vi "Select Channels Dialog.vi"(7 "Channel Label":string="System Channels", 8 "error in (no error)":errorcluster, 9 "Custom Filter":refnum<k24>, 10 "Filter":u8(ring)=1 items=["K_CHAN_R", "K_CHAN_W", "K_CHAN_RW", "K_CHAN_VOLT", "K_CHAN_FAULT", "K_ALL", "K_CUSTOM"], 11 "Start Item Ref":T1=18446744073709551615 format="%.0x") -> (0 "error out":errorcluster, 1 "Canceled":bool, 3 "Channels":string[](array[string]))   [LabVIEW 2013, in "Datadashboard CD Custom Device.lvlib"]
uses:
  Datadashboard CD Custom Device.lvlib
  <vilib>/NI Veristand/Custom Device API/Custom Device Item Ref.ctl
  NationalInstruments.VeriStand.SystemStorageUI
  NationalInstruments.VeriStand.SystemStorage
  <vilib>/NI Veristand/Custom Device API/Custom Device API.lvlib
panel:
  in  "OK":bool
  in  "Cancel":bool
  in  "TreeBrowserWF":refnum<k24>(container)
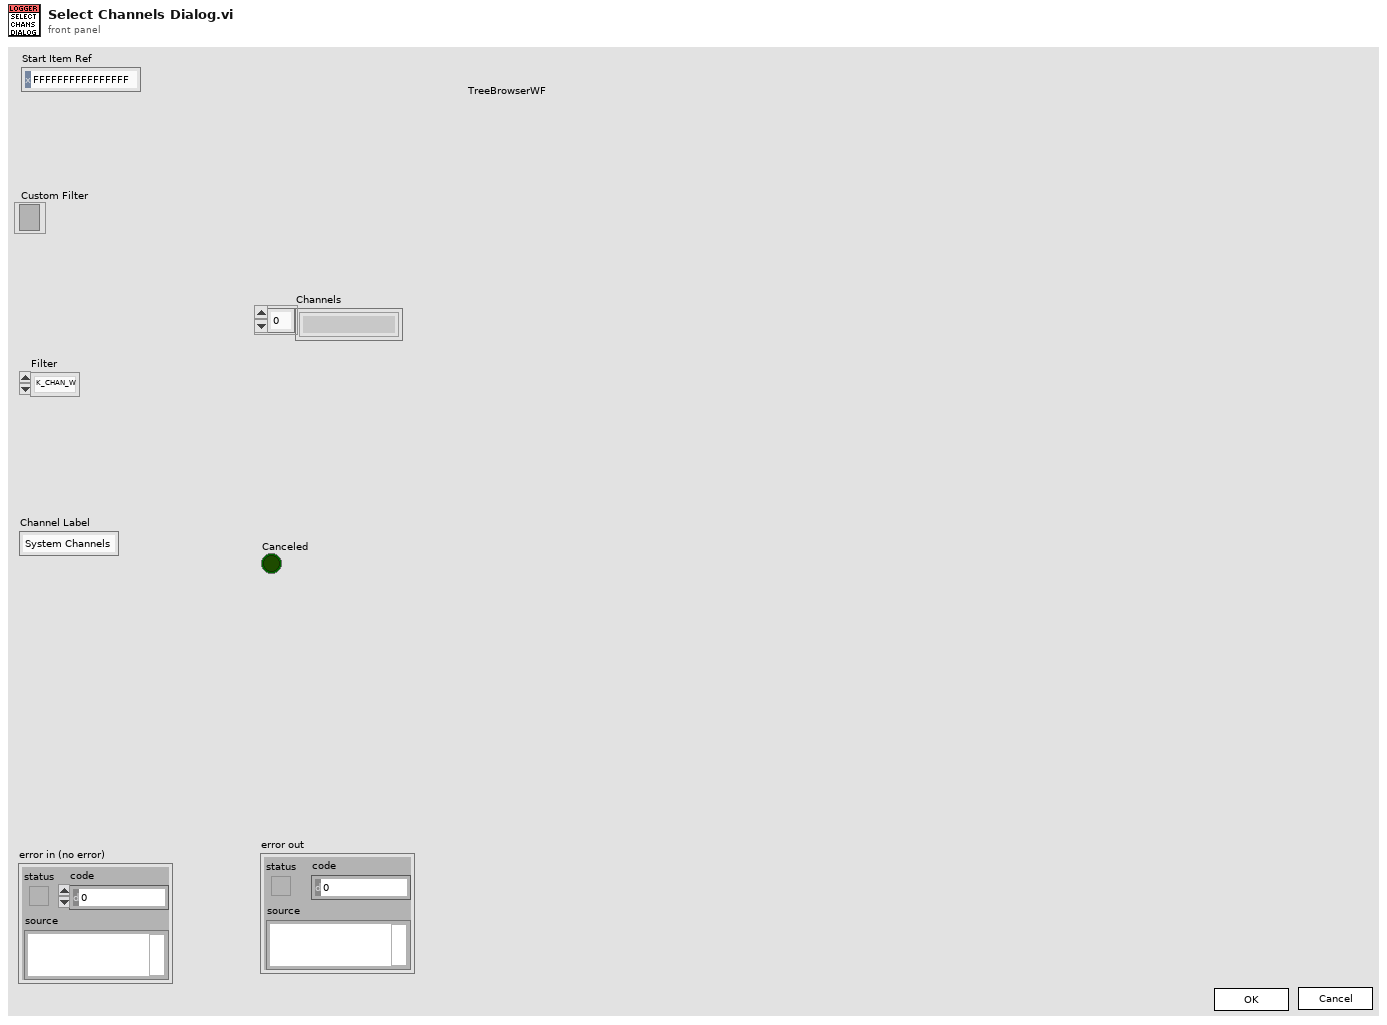
[diagram p1: front panel]
types:
  T1 = typedef "Custom Device API.lvlib/Custom Device Item Ref.ctl" = u64
  T2 = cluster{"Shut Down":bool, "Error":errorcluster, "Root":refnum<k24>, "Cancel":bool, "MapTree":cluster{"Ref":refnum<k24>, "Filter":refnum<k24>}, "Channels":string[]}
  T3 = typedef "Custom Device API.lvlib/Custom Device Pointer.ctl" = refnum<k24>
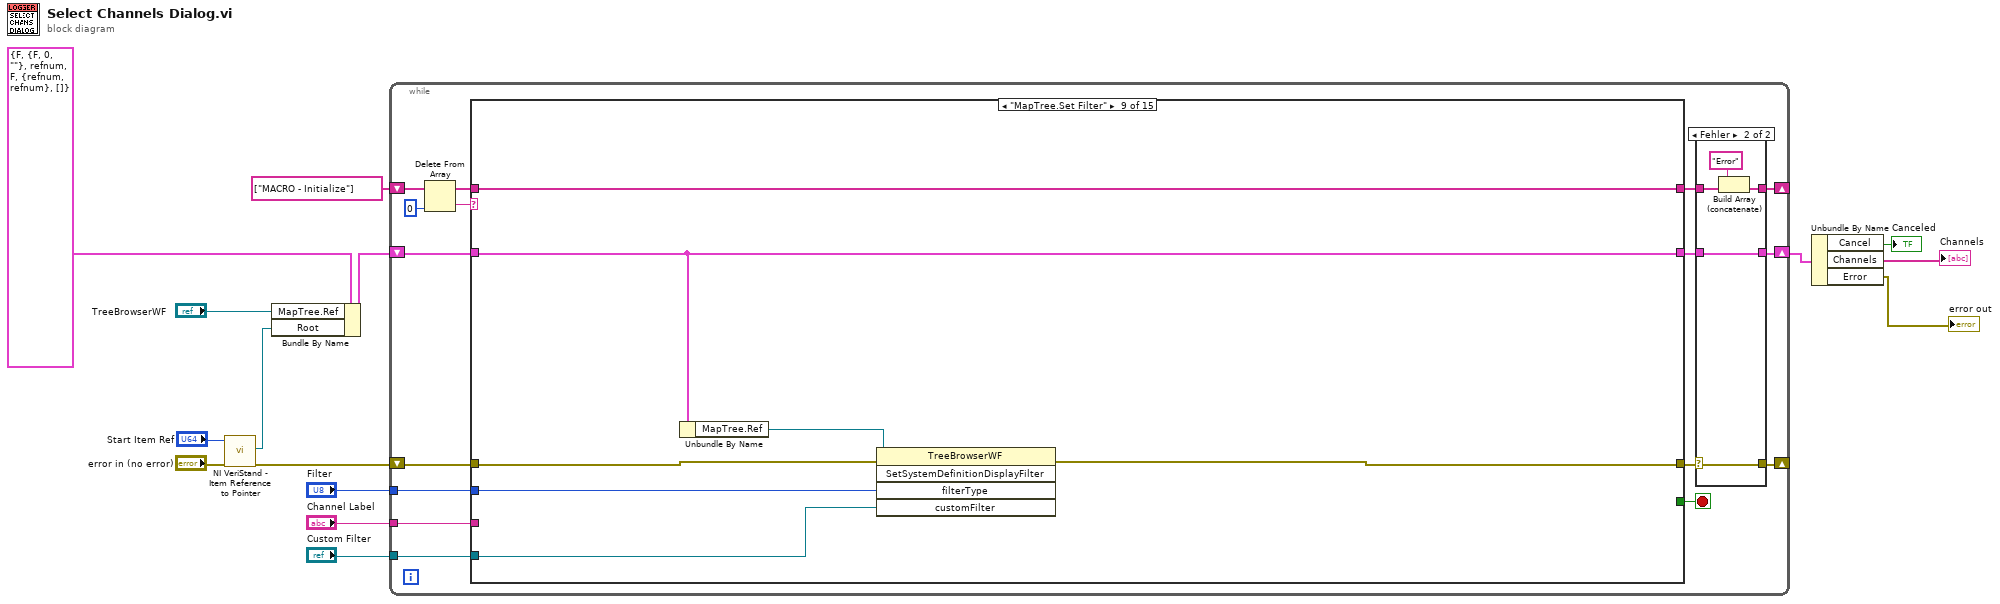
[diagram p0: block diagram]
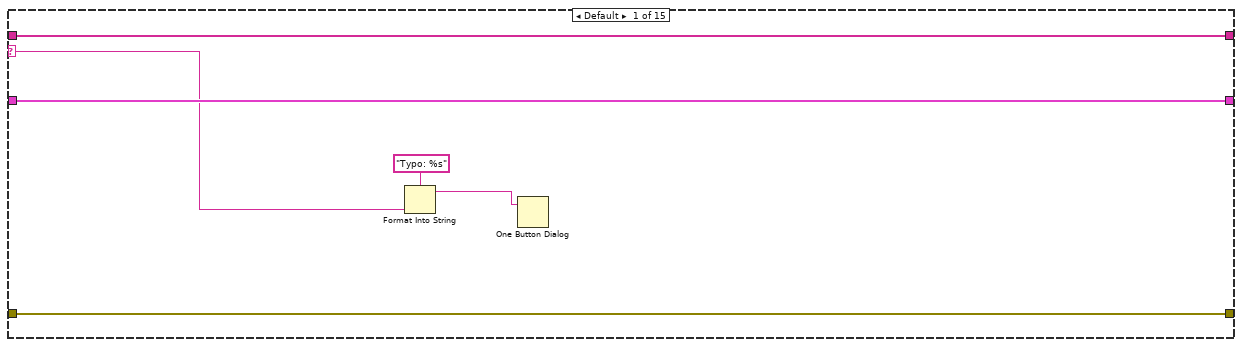
[diagram p3: hidden frame]
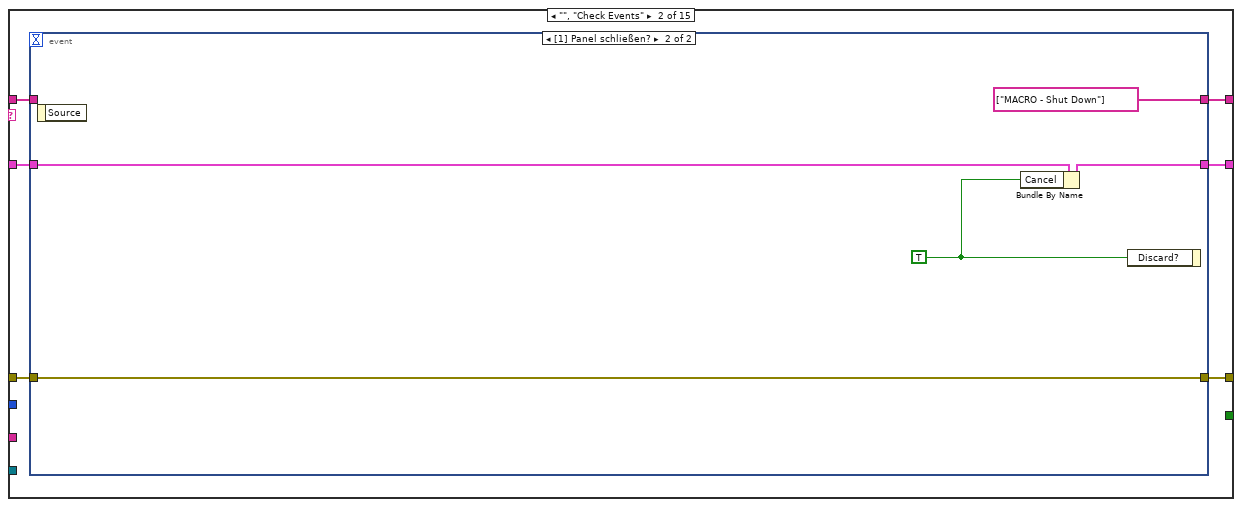
[diagram p4: hidden frame]
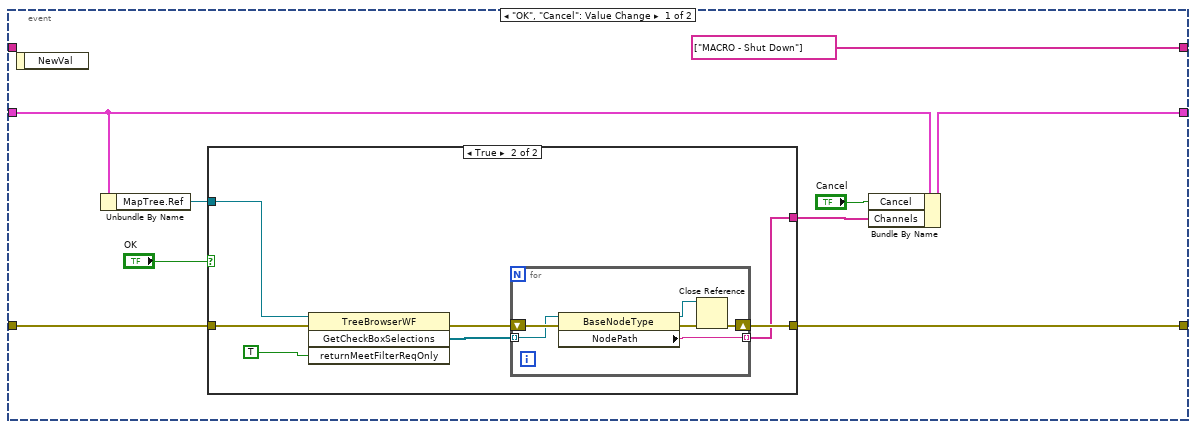
[diagram p5: hidden frame]
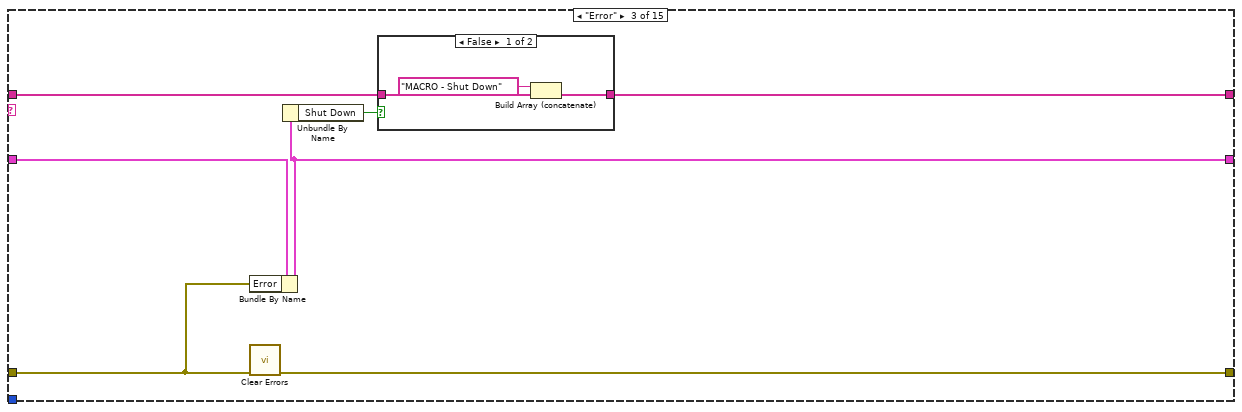
[diagram p7: hidden frame]
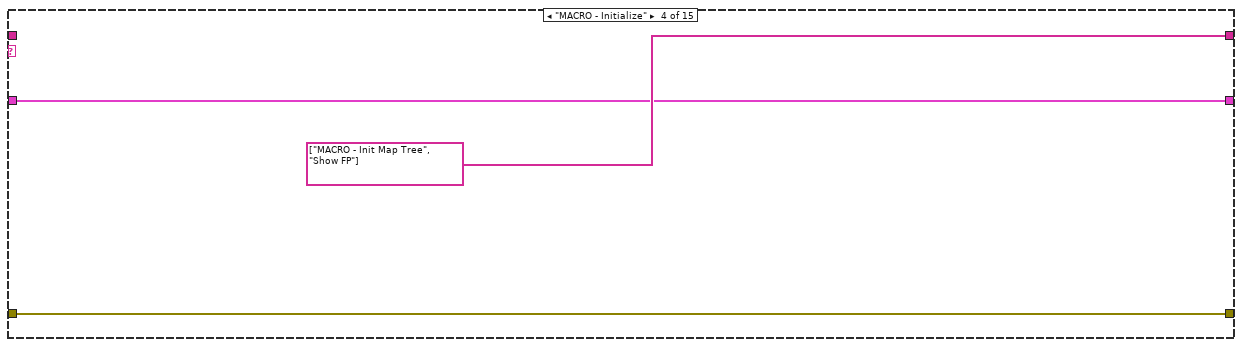
[diagram p9: hidden frame]
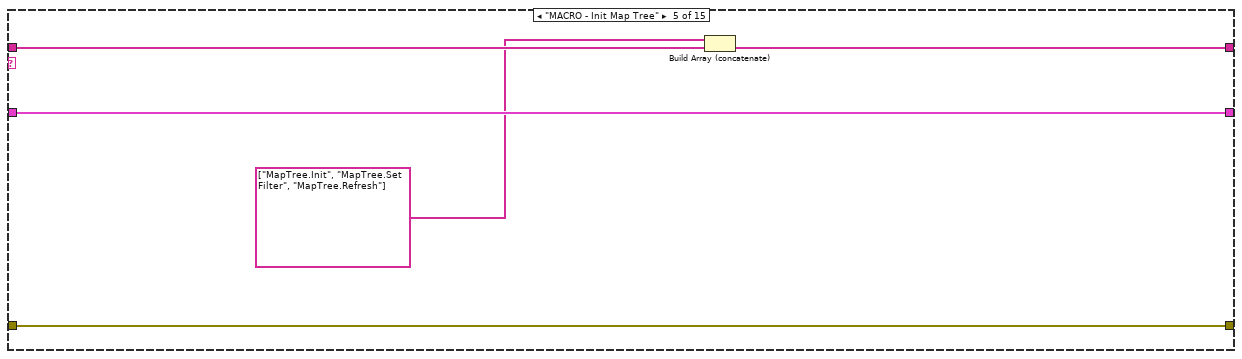
[diagram p10: hidden frame]
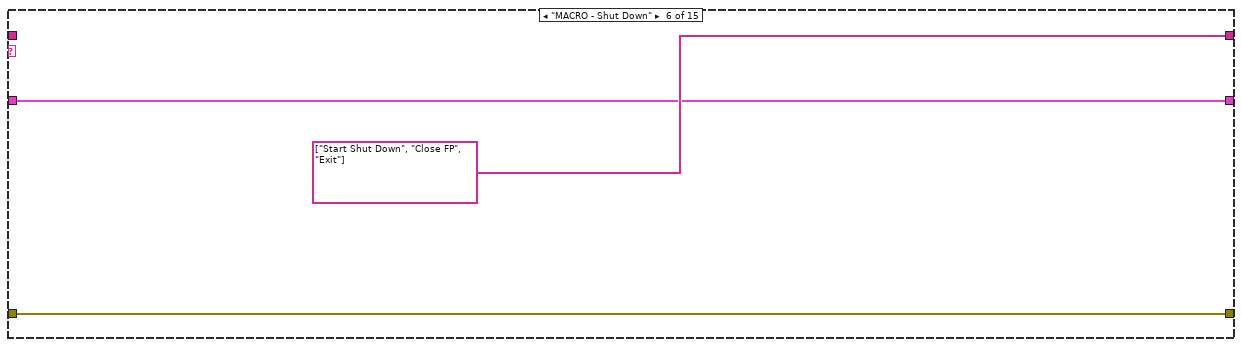
[diagram p11: hidden frame]
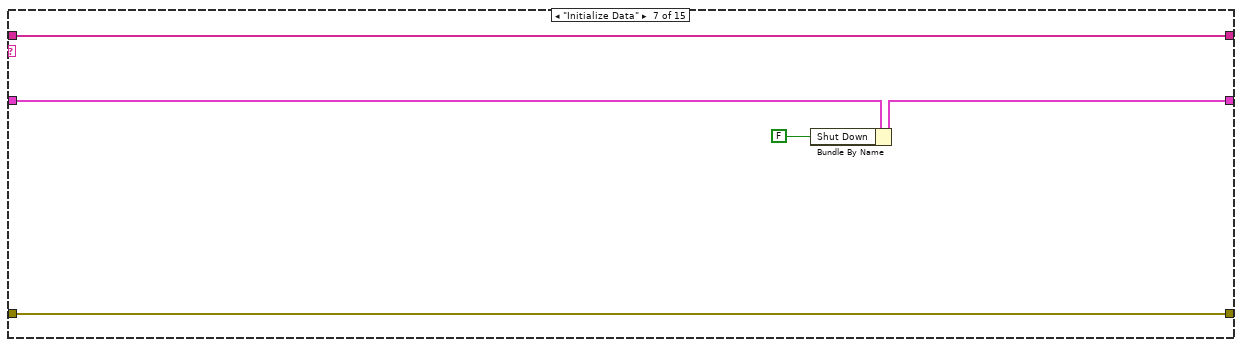
[diagram p12: hidden frame]
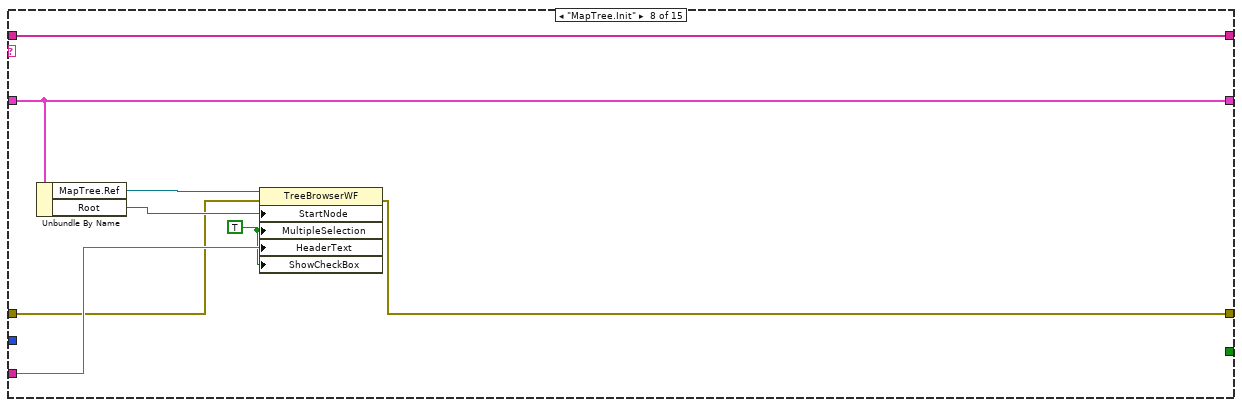
[diagram p13: hidden frame]
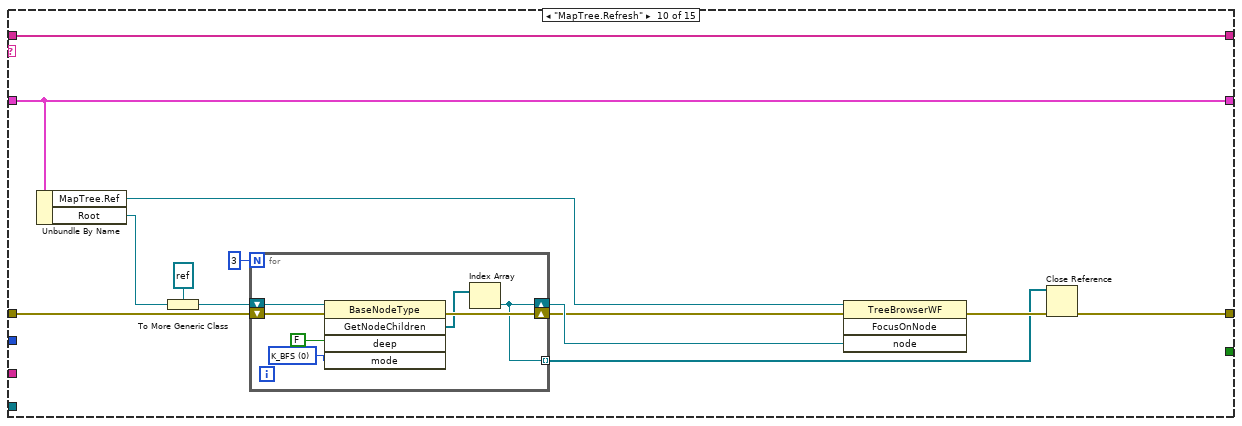
[diagram p14: hidden frame]
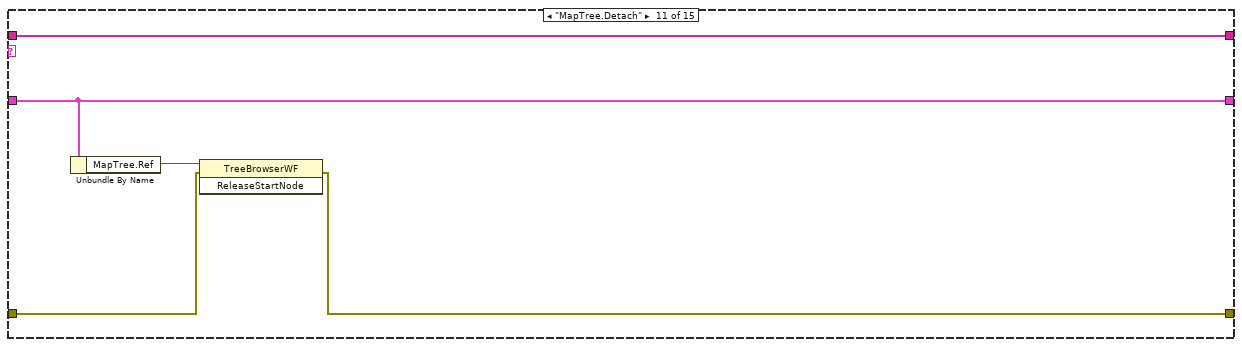
[diagram p15: hidden frame]
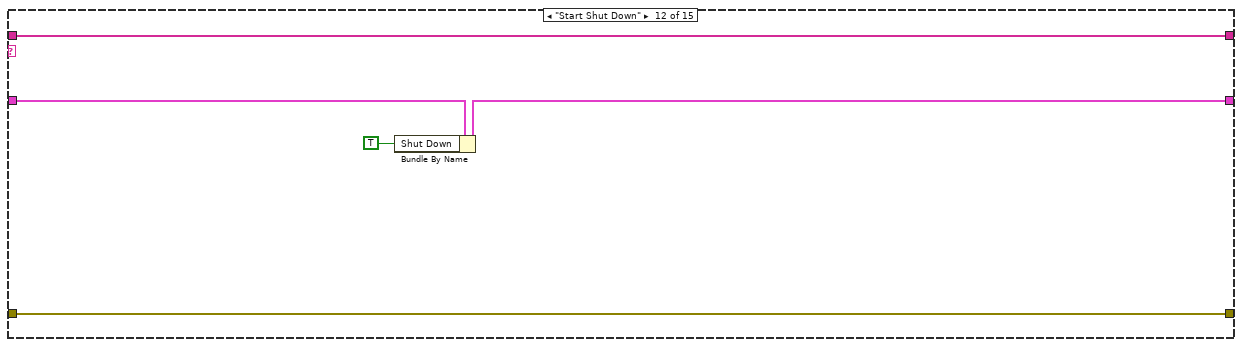
[diagram p16: hidden frame]
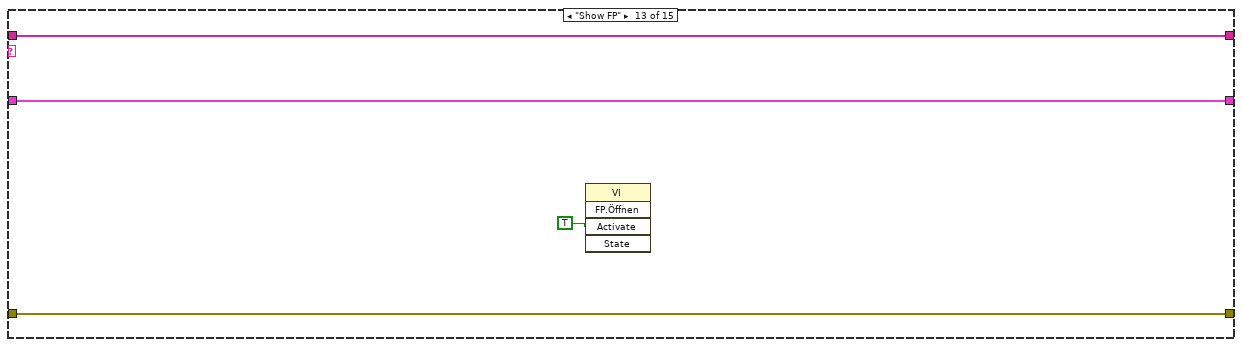
[diagram p17: hidden frame]
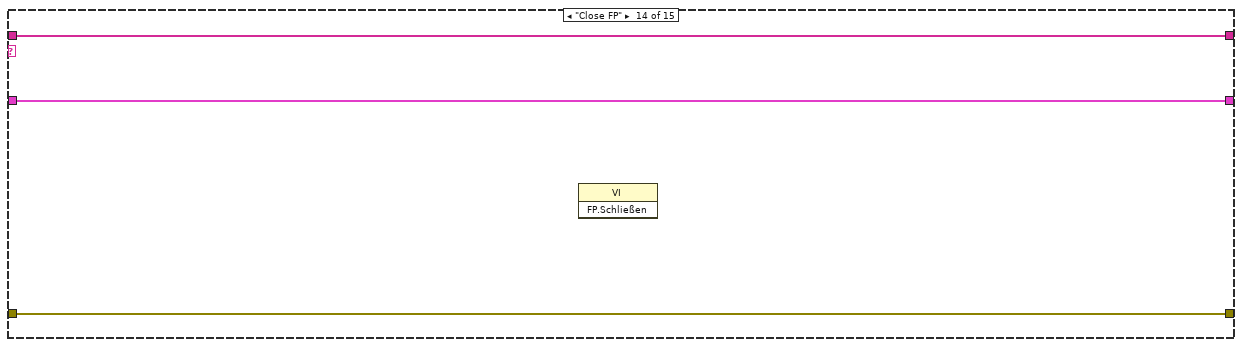
[diagram p18: hidden frame]
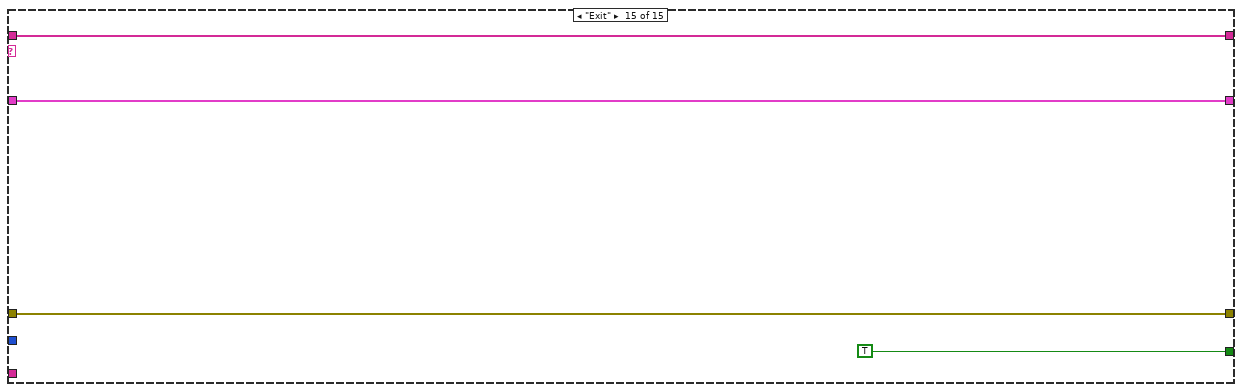
[diagram p19: hidden frame]
diagram:
  n1 = call <vilib>:"NI VeriStand - Item Reference to Pointer.vi"("error in (no error)"="error in (no error)", "Item Ref in"="Start Item Ref") -> ("error out"=w1:errorcluster, "Node Pointer"=w3:T3)  [unwired: 6 in, 2 out]
  n2 = Bundle By Name(cluster=T2 {"Shut Down"=FALSE, "Error"={"status"=FALSE, "code"=0, "source"=""}, "Root"=refnum, "Cancel"=FALSE, "MapTree"={"Ref"=refnum, "Filter"=refnum}, "Channels"=[]} ("State Data"), "MapTree.Ref"="TreeBrowserWF", "Root"=w3) -> (w12:T2)
  n3 = while {
    shift-right: [w21] -> _
    shift-left: string[] ["MACRO - Initialize"] -> [w31]
    shift-right: [w23] -> _
    shift-left: w1 -> [w27]
    shift-right: [w20] -> w8
    shift-left: w12 -> [w25]
    tunnel: "Channel Label" -> [w18]
    tunnel: "Filter" -> [w17]
    tunnel: "Custom Filter" -> [w16]
    stop <- w26 stop-if-true
    n4 = Delete From Array(array=w31, index=0) -> (deleted portion=w28:string, array with subset deleted=w29:string[])  [unwired: 1 in]
    n5 = case shown="\"MapTree.Set Filter\"" w28 {
      selector: w28 -> [w41 _ _ _ _ _ _ _ _ _ _ _ _ _ _]
      tunnel: w29 -> [w45 w51 w83 _ w98 _ w106 w114 w121 w134 w146 w147 w155 w158 w162]
      tunnel: [w45 w46 w82 string[] ["MACRO - Init Map Tree", "Show FP"] ("array") w95 string[] ["Start Shut Down", "Close FP", "Exit"] ("array") w106 w114 w121 w134 w146 w147 w155 w158 w162] -> w22
      tunnel: [w44 w49 w80 w93 w97 w101 w105 w107 w119 w124 w142 w151 w154 w157 w161] -> w24
      tunnel: w27 -> [w44 w48 w81 w93 w97 w101 w105 w108 w117 w132 w143 w151 w154 w157 w161]
      tunnel: [_ _ _ _ _ _ _ _ _ _ _ _ _ _ TRUE] -> w26
      tunnel: w25 -> [w43 w50 w86 w91 w96 w99 w102 w113 w118 w133 w145 w150 w153 w156 w159]
      tunnel: [w43 w47 w85 w91 w96 w99 w104 w113 w118 w133 w145 w149 w153 w156 w159] -> w19
      tunnel: w18 -> [_ _ _ _ _ _ _ w110 _ _ _ _ _ _ _]
      tunnel: w17 -> [_ _ _ _ _ _ _ _ w116 _ _ _ _ _ _]
      tunnel: w16 -> [_ _ _ _ _ _ _ _ w115 _ _ _ _ _ _]
      frame Default {
        n6 = Format Into String(format string="Typo: %s", w41) -> (resulting string=w40:string)  [unwired: 2 in, 1 out]
        n7 = One Button Dialog(message=w40) -> ()  [unwired: 1 in, 1 out]
      }
      frame "", "Check Events" {
        n8 = event shown="[1] Panel schließen?" {
          selector: _ -> [_ _]
          dyn-events: _ -> [_ _]
          timeout: _ -> [_ _]
          tunnel: [w53 w79] -> w49
          tunnel: w48 -> [w55 w79]
          tunnel: [w59 w76] -> w47
          tunnel: w50 -> [w57 w78]
          tunnel: w51 -> [_ _]
          tunnel: [string[] ["MACRO - Shut Down"] string[] ["MACRO - Shut Down"]] -> w46
          event "OK", "Cancel": Value Change {
            n9 = event-data() -> ()  [unwired: 1 in, 1 out]
            n10 = Unbundle By Name(w57) -> ("MapTree.Ref"=w56:refnum<k24>)
            n11 = case shown="True" "OK" {
              tunnel: w56 -> [_ w68]
              tunnel: w55 -> [w61 w67]
              tunnel: [_ w62] -> w54
              tunnel: [w61 w63] -> w53
              frame False {
              }
              frame True {
                n12 = invoke class="TreeBrowserWF" method="GetCheckBoxSelections"(reference=w68, error in=w67, "returnMeetFilterReqOnly"=TRUE) -> (error out=w65:errorcluster, "GetCheckBoxSelections"=w64:refnum<k24>[])  [unwired: 1 in, 2 out]
                n13 = for {
                  shift-right: [w69] -> w63
                  shift-left: w65 -> [w74]
                  tunnel: w64 -> [w73] mode=indexing
                  tunnel: [w72] -> w62 mode=indexing
                  n14 = property class="BaseNodeType"(reference=w73, error in=w74) -> (reference out=w70:refnum<k24>, error out=w71:errorcluster, "NodePath"=w72:string)
                  n15 = Close Reference(reference=w70, error in (no error)=w71) -> (error out=w69:errorcluster)
                }
              }
            }
            n16 = Bundle By Name(cluster=w57, "Cancel"="Cancel", "Channels"=w54) -> (w59:T2)
          }
          event Panel Close? {
            w75 = TRUE ("Discard?")
            n17 = event-data() -> ()  [unwired: 1 in, 1 out]
            n18 = Bundle By Name(cluster=w78, "Cancel"=w75) -> (w76:T2)
            n19 = event-data("Discard?"=w75) -> ()  [unwired: 1 in, 1 out]
          }
        }
      }
      frame "Error" {
        n20 = Bundle By Name(cluster=w86, "Error"=w81) -> (w85:T2)
        n21 = call <vilib>:"Clear Errors.vi"("error in (no error)"=w81) -> ("error out"=w80:errorcluster)  [unwired: 6 in]
        n22 = Unbundle By Name(w85) -> ("Shut Down"=w84:bool)
        n23 = case shown="False" w84 {
          tunnel: w83 -> [w88 w90]
          tunnel: [w87 w90] -> w82
          frame False {
            n24 = Build Array (concatenate)("MACRO - Shut Down", w88) -> (w87:string[])
          }
          frame True {
            # "Do not interrupt a shut down sequence. This can cause an infinite loop."
          }
        }
      }
      frame "MACRO - Initialize" {
      }
      frame "MACRO - Init Map Tree" {
        n25 = Build Array (concatenate)(string[] ["MapTree.Init", "MapTree.Set Filter", "MapTree.Refresh"] ("array"), w98) -> (w95:string[])
      }
      frame "MACRO - Shut Down" {
      }
      frame "Initialize Data" {
        n26 = Bundle By Name(cluster=w102, "Shut Down"=FALSE) -> (w104:T2)
      }
      frame "MapTree.Init" {
        w109 = TRUE ("MultipleSelection")
        n27 = Unbundle By Name(w113) -> ("MapTree.Ref"=w112:refnum<k24>, "Root"=w111:refnum<k24>)
        n28 = property class="TreeBrowserWF"(reference=w112, error in=w108, "StartNode"=w111, "MultipleSelection"=w109, "HeaderText"=w110, "ShowCheckBox"=w109) -> (error out=w107:errorcluster)  [unwired: 1 out]
      }
      frame "MapTree.Set Filter" {
        n29 = Unbundle By Name(w118) -> ("MapTree.Ref"=w120:refnum<k24>)
        n30 = invoke class="TreeBrowserWF" method="SetSystemDefinitionDisplayFilter"(reference=w120, error in=w117, "filterType"=w116, "customFilter"=w115) -> (error out=w119:errorcluster)  [unwired: 1 in, 4 out]
      }
      frame "MapTree.Refresh" {
        n31 = Unbundle By Name(w133) -> ("MapTree.Ref"=w122:refnum<k24>, "Root"=w131:refnum<k24>)
        n32 = To More Generic Class(target class=refnum<k24> refnum, reference=w131) -> (generic class reference=w129:refnum<k24>)
        n33 = for {
          N: 3 -> [_]
          shift-right: [w135] -> w128
          shift-left: w129 -> [w138]
          shift-right: [w141] -> w123
          shift-left: w132 -> [w137]
          tunnel: [w135] -> w125 mode=indexing
          w139 = 0 items=["K_BFS", "K_DFS", "K_CHILDONLY", "K_UP"] ("mode")
          n34 = invoke class="BaseNodeType" method="GetNodeChildren"(reference=w138, error in=w137, "deep"=FALSE, "mode"=w139) -> (error out=w141:errorcluster, "GetNodeChildren"=w136:refnum<k24>[])  [unwired: 1 in, 3 out]
          n35 = Index Array(array=w136) -> (element=w135:refnum<k24>)  [unwired: 1 in]
        }
        n36 = invoke class="TreeBrowserWF" method="FocusOnNode"(reference=w122, error in=w123, "node"=w128) -> (error out=w126:errorcluster)  [unwired: 1 in, 3 out]
        n37 = Close Reference(reference=w125, error in (no error)=w126) -> (error out=w124:errorcluster)
      }
      frame "MapTree.Detach" {
        n38 = Unbundle By Name(w145) -> ("MapTree.Ref"=w144:refnum<k24>)
        n39 = invoke class="TreeBrowserWF" method="ReleaseStartNode"(reference=w144, error in=w143) -> (error out=w142:errorcluster)  [unwired: 1 in, 2 out]
      }
      frame "Start Shut Down" {
        n40 = Bundle By Name(cluster=w150, "Shut Down"=TRUE) -> (w149:T2)
      }
      frame "Show FP" {
        n41 = invoke class="VI" method="FP.Öffnen"("Activate"=TRUE ("Activate?")) -> ()  [unwired: 4 in, 5 out]
      }
      frame "Close FP" {
        n42 = invoke class="VI" method="FP.Schließen"() -> ()  [unwired: 3 in, 3 out]
      }
      frame "Exit" {
      }
    }
    n43 = case shown="Fehler" w24 {
      selector: w24 -> [w34 w39]
      tunnel: [w34 w39] -> w23
      tunnel: w22 -> [w33 w37]
      tunnel: [w33 w36] -> w21
      tunnel: [w32 w38] -> w20
      tunnel: w19 -> [w32 w38]
      frame No Error {
      }
      frame Error {
        n44 = Build Array (concatenate)("Error", w37) -> (w36:string[])
      }
    }
  }
  n45 = Unbundle By Name(w8) -> ("Cancel"=→"Canceled":bool, "Channels"=→"Channels":string[], "Error"=→"error out":errorcluster)
